vi "Main.vi"() -> ()   [LabVIEW 2015]
doc: "The myRIO Project template acquires acceleration data from the onboard accelerometer and displays the changes of acceleration values in a waveform chart."
uses:
  <vilib>/myRIO/Instrument Drivers/Onboard IO/UART/typedef/VISA Configuration.ctl
  <vilib>/Instr/_visa.llb/VISA Configure Serial Port (Instr).vi
  <vilib>/myRIO/Express VI/Onboard IO/UART/UART Express VI.xnode
  <vilib>/myRIO/Instrument Drivers/Onboard IO/UART/UART.lvlib
panel:
  out "Measured Resistance":u32
  out "Ambient Temperature":dbl
  in  "Stop Button":bool
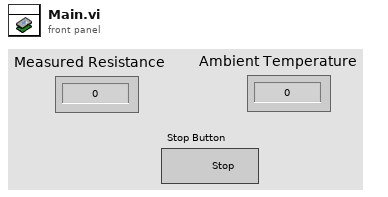
[diagram p1: front panel]
types:
  T1 = typedef "UART.lvlib/VISA Configuration.ctl" = cluster{"baud rate (9600)":u32, "data bits (8)":u16, "parity (0:none)":enum16{"None", "Odd", "Even", "Mark", "Space"}, "stop bits (10: 1 bit)":u16, "flow control (0:none)":u16, "termination char\n(0xA = '\\n' = LF) ":u8, "Enable Termination\nChar (T)":bool, "timeout (10sec)":u32}
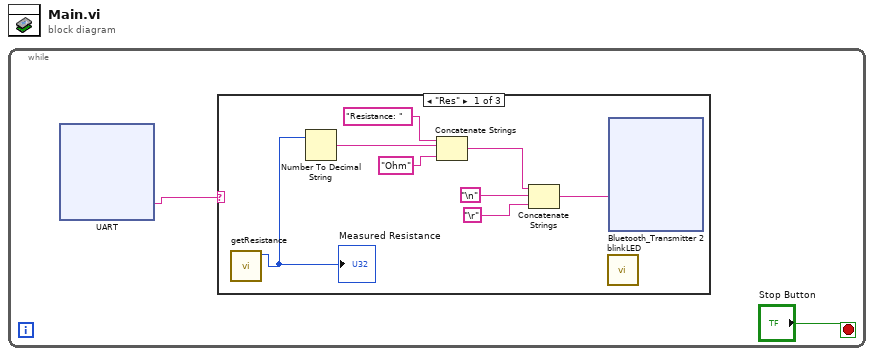
[diagram p0: block diagram]
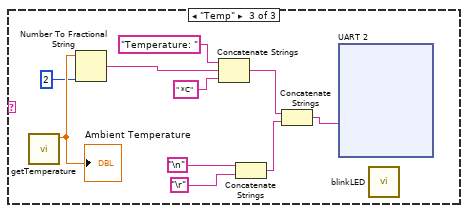
[diagram p3: hidden frame]
diagram:
  n1 = while {
    stop <- "Stop Button" stop-if-true
    n2 = xnode "UART"() -> ("Characters Read"=w1:string)  [unwired: 1 in, 1 out]
    n3 = case shown="\"Res\"" w1 {
      frame "Res" {
        n4 = call "getResistance.vi"() -> ("Measured Resistance"=w4:u32)  [unwired: 11 in]
        "Measured Resistance" <- w4
        n5 = Number To Decimal String(number=w4) -> (decimal integer string=w5:string)  [unwired: 1 in]
        n6 = Concatenate Strings("Resistance: " ("string"), w5, "Ohm" ("string")) -> (w7:string)
        n7 = Concatenate Strings(w7, "\n", "\r") -> (w8:string)
        n8 = call "blinkLED.vi"() -> ()  [unwired: 12 in]
        n9 = xnode "Bluetooth_Transmitter 2"("Characters to Write"=w8) -> ()  [unwired: 1 in, 2 out]
      }
      frame Default {
      }
      frame "Temp" {
        n10 = call "getTemperature.vi"() -> ("Measured Temperature [*C]"=w32:dbl)  [unwired: 10 in, 1 out]
        "Ambient Temperature" <- w32
        n11 = Number To Fractional String(number=w32, precision (6)=i16 2 ("width (-)")) -> (F-format string=w29:string)  [unwired: 2 in]
        n12 = Concatenate Strings("Temperature: ", w29, " *C" ("string")) -> (w27:string)
        n13 = Concatenate Strings("\n", "\r") -> (w34:string)
        n14 = Concatenate Strings(w27, w34) -> (w33:string)
        n15 = xnode "UART 2"("Characters to Write"=w33) -> ()  [unwired: 1 in, 2 out]
        n16 = call "blinkLED.vi"() -> ()  [unwired: 12 in]
      }
    }
  }
